vi "ReadDictionary.vi"(8 "error in (no error)":errorcluster, 11 "Dictionary File Path":path) -> (0 "error out":errorcluster, 1 "ASCII String":string, 2 "Dictionary":T1, 3 "Dictionary File Path out":path)   [LabVIEW 2017, in "JKI Simple Localization.lvlib"]
uses:
  API/JKI Simple Localization.lvlib
  Definitions/Dictionary--Cluster.ctl
  Definitions/Private/Font -- Cluster.ctl
  Definitions/Private/Phrase Dictionary Entry -- Cluster.ctl
  <vilib>/addons/_JKI.lib/Serialization/JSON/JKI JSON Serialization.lvlib
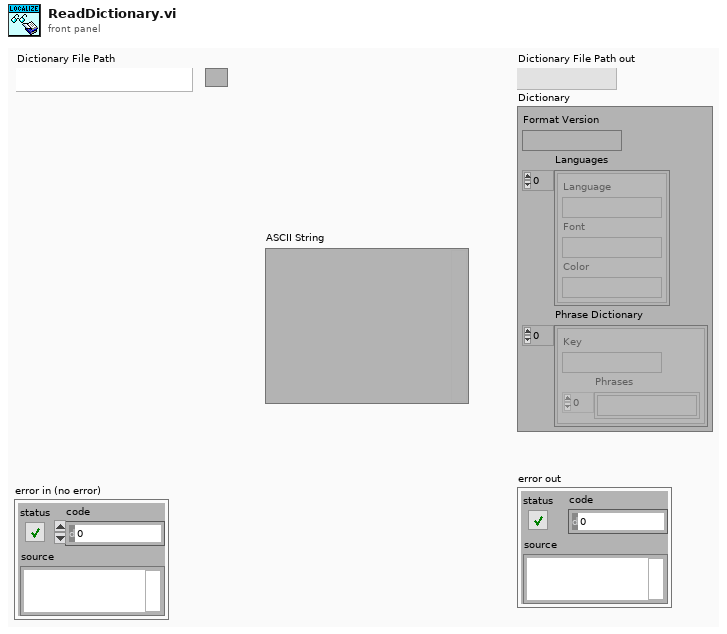
[diagram p1: front panel]
types:
  T1 = typedef "JKI Simple Localization.lvlib/Dictionary--Cluster.ctl" = cluster{"Format Version":string, "Languages":T2[], "Phrase Dictionary":T3[]}
  T2 = typedef "JKI Simple Localization.lvlib/Font -- Cluster.ctl" = cluster{"Language":string, "Font":string, "Color":string}
  T3 = typedef "JKI Simple Localization.lvlib/Phrase Dictionary Entry -- Cluster.ctl" = cluster{"Key":string, "Phrases":string[]}
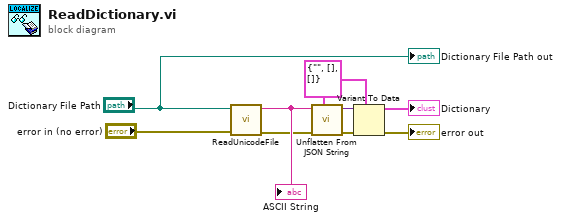
[diagram p0: block diagram]
diagram:
  w2 = T1 {"Format Version"="", "Languages"=[], "Phrase Dictionary"=[]} ("Localization")
  n1 = call "ReadUnicodeFile.vi"("error in (no error)"="error in (no error)", "Unicode File Path"="Dictionary File Path") -> ("error out"=w6:errorcluster, "ASCII String"=w7:string)  [unwired: 8 in]
  "ASCII String" <- w7
  n2 = call <vilib>:"Unflatten From JSON String.vi"("Type and Defaults"=w2, "error in (no error)"=w6, "JSON String"=w7) -> ("error out"=w4:errorcluster, "Variant"=w5:variant)  [unwired: 7 in]
  n3 = Variant To Data(error in=w4, type=w2, Variant=w5) -> (data=→"Dictionary":T1, error out=→"error out":errorcluster)
  "Dictionary File Path out" <- "Dictionary File Path"
